vi "TCP_finding.vi"() -> ()   [LabVIEW 2018]
uses:
  <vilib>/Platform/TimedLoop/XDataNode/timing_clust.ctl
  <vilib>/Platform/TimedLoop/XDataNode/nitl_modes.ctl
  <vilib>/Platform/TimedLoop/XDataNode/wakeup.ctl
  <vilib>/Analysis/_algsub.llb/Real PseudoInverse Matrix.vi
  <vilib>/Analysis/baseanly.llb/A x Vector.vi
  <vilib>/Analysis/Matrix/Numeric/Subtract/Subtract - RM,RM.vi
  <vilib>/Platform/TimedLoop/XDataNode/XDataNode.xnode
  <vilib>/Platform/TimedLoop/XDataNode/XDNodeRunTimeDep.lvlib
  <vilib>/Analysis/Matrix/NI_Matrix.lvlib
  <vilib>/Analysis/NI_AALPro.lvlib
  <vilib>/Analysis/NI_AALBase.lvlib
panel:
  in  "Set":bool
  out "Finished Late_Monitor":u32
  out "Finished Late_Matrix":u32
  in  "stop":bool
  out "Pos 3":T1={"X"=196.167, "Y"=47.983, "Z"=275.578, "X_theta"=160.982, "Y_theta"=40.126, "Z_theta"=-130.827} {"Z_theta" format="%#_8f"; "Y_theta" format="%#_8f"; "X_theta" format="%#_8f"; "Z" format="%#_8f"; "Y" format="%#_8f"; "X" format="%#_8f"}
  out "Pos 4":T1={"X"=168.527, "Y"=22.423, "Z"=245.207, "X_theta"=177.832, "Y_theta"=63.314, "Z_theta"=-166.919} {"Z_theta" format="%#_8f"; "Y_theta" format="%#_8f"; "X_theta" format="%#_8f"; "Z" format="%#_8f"; "Y" format="%#_8f"; "X" format="%#_8f"}
  out "Pos 2":T1={"X"=193.917, "Y"=-20.843, "Z"=266.17, "X_theta"=-149.895, "Y_theta"=42.769, "Z_theta"=158.347} {"Z_theta" format="%#_8f"; "Y_theta" format="%#_8f"; "X_theta" format="%#_8f"; "Z" format="%#_8f"; "Y" format="%#_8f"; "X" format="%#_8f"}
  out "Pos 1":T1={"X"=173.917, "Y"=16.457, "Z"=254.971, "X_theta"=-176.204, "Y_theta"=57.893, "Z_theta"=-177.155} {"Z_theta" format="%#_8f"; "Y_theta" format="%#_8f"; "X_theta" format="%#_8f"; "Z" format="%#_8f"; "Y" format="%#_8f"; "X" format="%#_8f"}
  out "TCP":dbl[](array[numeric]) format="%#_4g"
  in  "find":bool
  in  "Save Pos 4":bool
  in  "Save Pos 3":bool
  in  "Save Pos 2":bool
  in  "Save Pos 1":bool
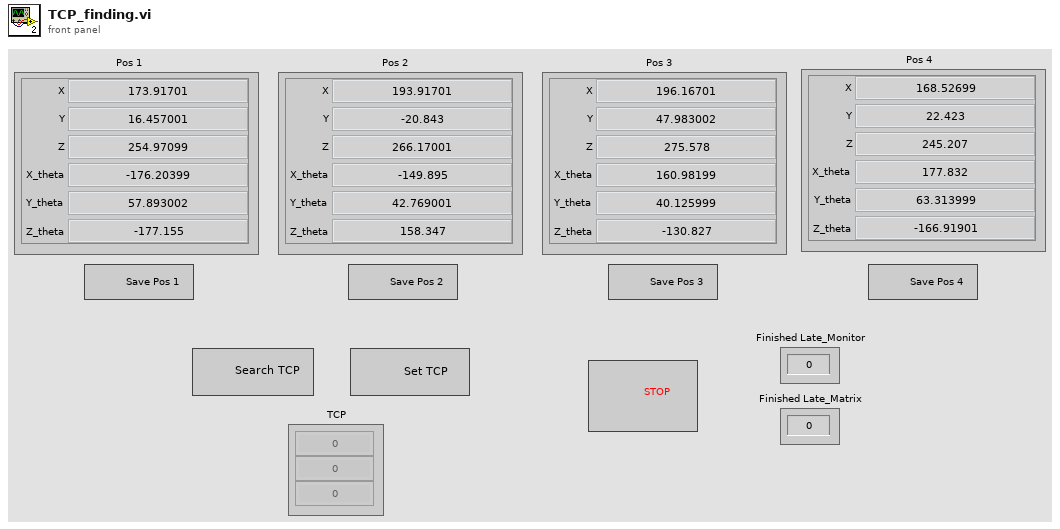
[diagram p1: front panel]
types:
  T1 = cluster{"X":sgl, "Y":sgl, "Z":sgl, "X_theta":sgl, "Y_theta":sgl, "Z_theta":sgl}
  T2 = typedef "XDNodeRunTimeDep.lvlib/timing_clust.ctl" = cluster{"Expected End [f-1]":u64, "Actual End [f-1]":u64, "Finished Late? [f-1]":bool, "Expected End [i-1]":u64, "Actual End [i-1]":u64, "Finished Late? [i-1]":bool, "Expected Start [i]":u64, "Actual Start [i]":u64, "Expected Start [f]":u64, "Actual Start [f]":u64, "Source Name":string, "Structure Name":string, "Period":i64, "Deadline":i64, "Offset":i64, "Start":i64, "Priority":i32, "Timeout":i32, "Mode":T3, "Wakeup Reason":T4, "Error":errorcluster, "Source Type":string, "Secondary Source Type":string, "Global End Time":u64, "Global Start Time":u64, "Frame Duration":u64, "Iteration Duration":u64, "Assigned CPU":i32, "I/O Scan Engine Mode":u32}
  T3 = typedef "XDNodeRunTimeDep.lvlib/nitl_modes.ctl" = enum32{"No Change", "Process missed periods, maintain original phase", "Discard missed periods, maintain original phase", "Process missed periods, ignore original phase", "Discard missed periods, ignore original phase"}
  T4 = typedef "XDNodeRunTimeDep.lvlib/wakeup.ctl" = enum32{"Normal", "Aborted", "Asynchronous wakeup", "Timing source error", "Timed loop error", "Timeout"}
  T5 = typedef "NI_Matrix.lvlib/RealMatrix.ctl" = dbl[][]
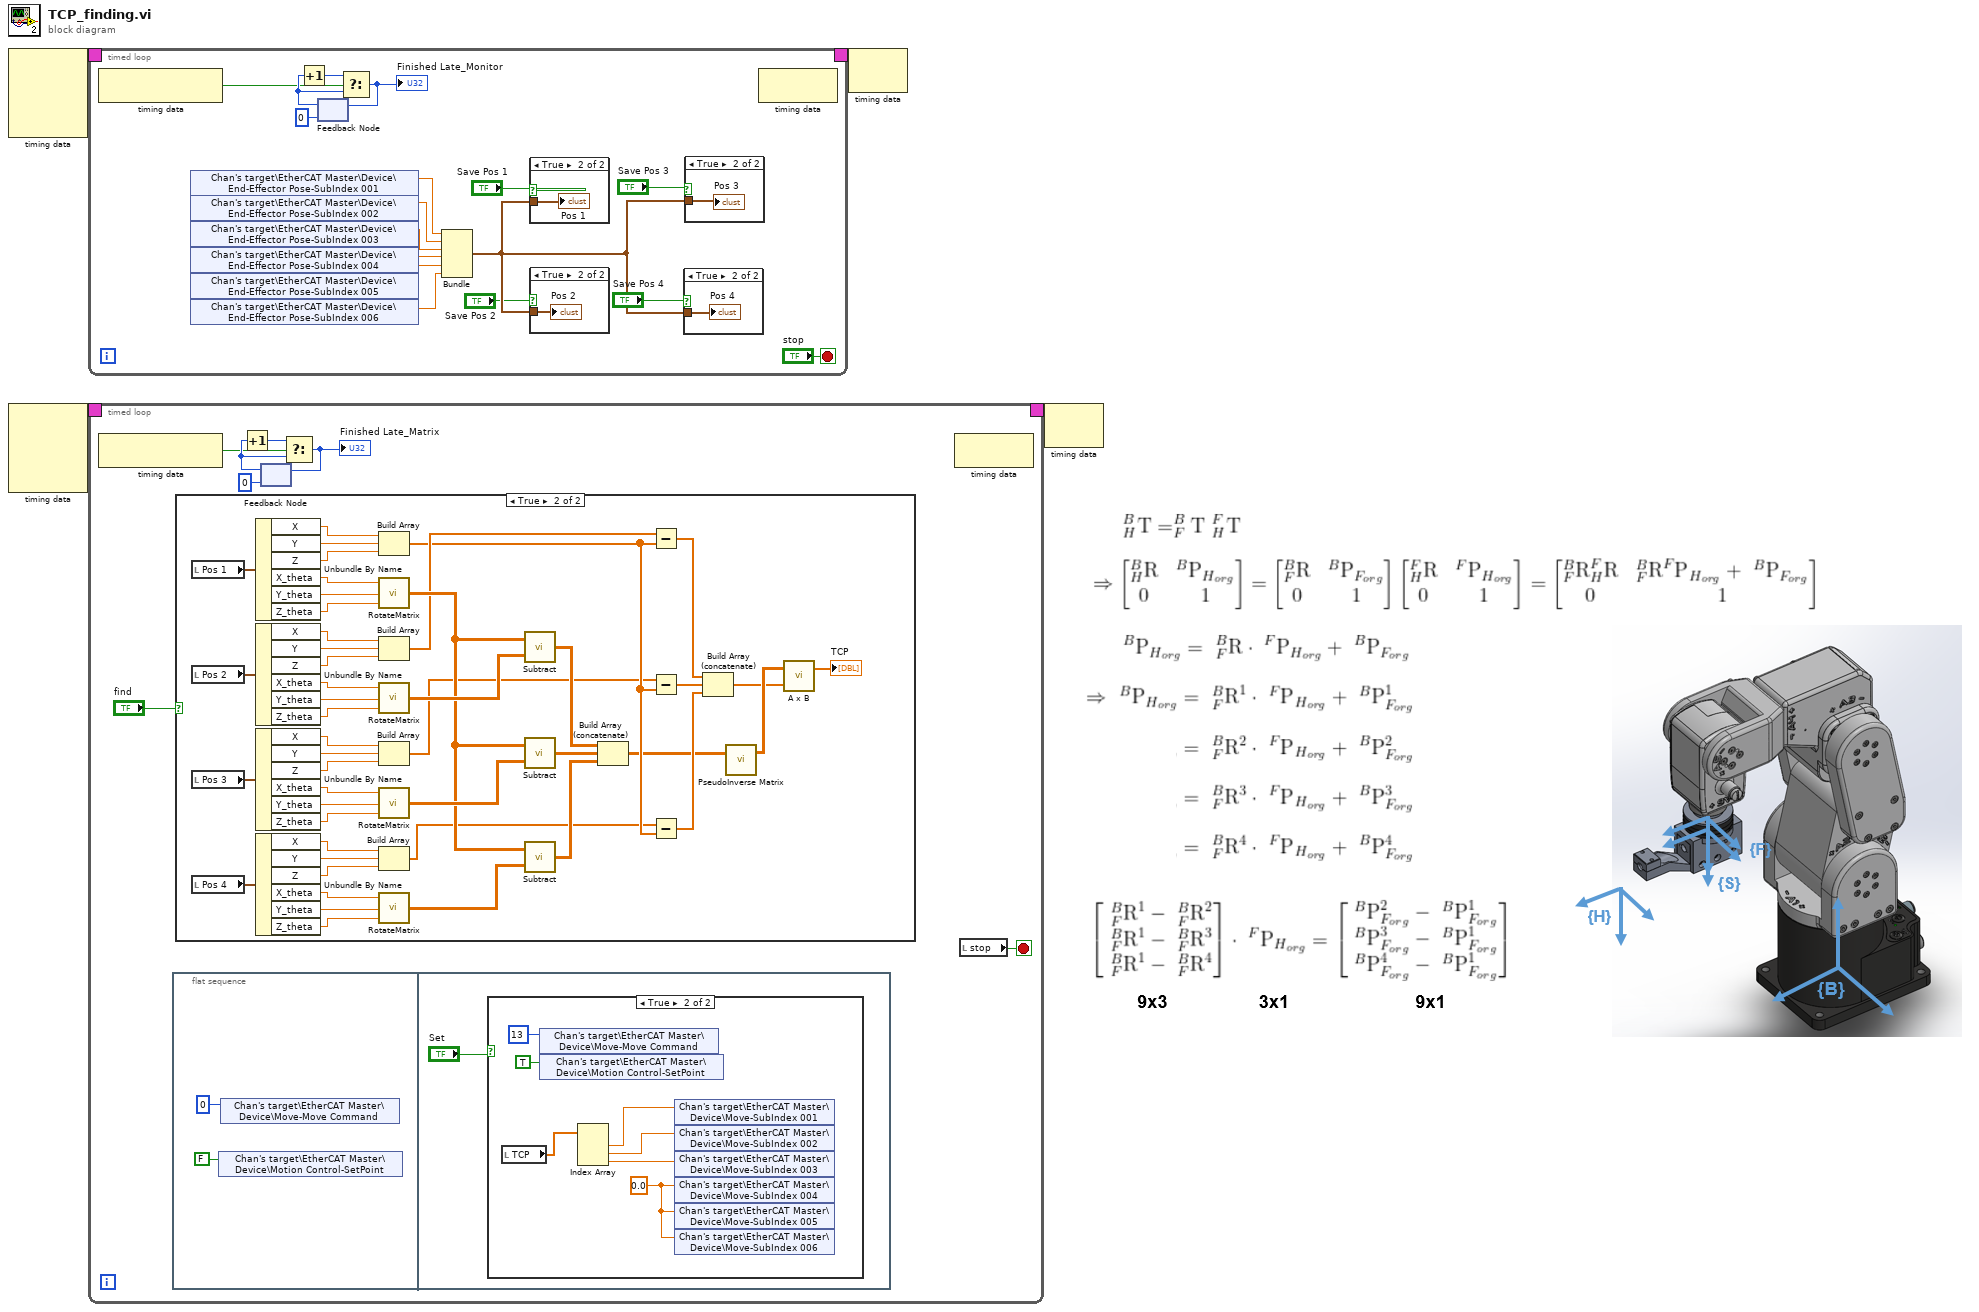
[diagram p0: block diagram]
diagram:
  n1 = node-c288() -> (w4:T2)  [unwired: 4 in]
  n2 = node-c288() -> (w2:T2)  [unwired: 4 in]
  n3 = timed-loop {
    timing: w4 -> [_]
    timing-out: [_] -> w3
    stop <- "stop" stop-if-true
    n4 = node-c288() -> (w5:bool)  [unwired: 1 in]
    n5 = shared-variable "Chan's target\\EtherCAT Master\\Device\\End-Effector Pose-SubIndex 001"() -> (w16:sgl)  [unwired: 1 in, 1 out]
    n6 = shared-variable "Chan's target\\EtherCAT Master\\Device\\End-Effector Pose-SubIndex 002"() -> (w17:sgl)  [unwired: 1 in, 1 out]
    n7 = shared-variable "Chan's target\\EtherCAT Master\\Device\\End-Effector Pose-SubIndex 003"() -> (w18:sgl)  [unwired: 1 in, 1 out]
    n8 = shared-variable "Chan's target\\EtherCAT Master\\Device\\End-Effector Pose-SubIndex 004"() -> (w19:sgl)  [unwired: 1 in, 1 out]
    n9 = shared-variable "Chan's target\\EtherCAT Master\\Device\\End-Effector Pose-SubIndex 005"() -> (w20:sgl)  [unwired: 1 in, 1 out]
    n10 = shared-variable "Chan's target\\EtherCAT Master\\Device\\End-Effector Pose-SubIndex 006"() -> (w21:sgl)  [unwired: 1 in, 1 out]
    n11 = feedback #1(u32 0) -> (w7:u32)
    n12 = Increment(x=w7) -> (x+1=w8:u32)
    n13 = Select(t=w8, s=w5, f=w7) -> (s? t:f=w9:u32)
    "Finished Late_Monitor" <- w9
    n14 = feedback-in #1(w9) -> ()
    n15 = Bundle(w16, w17, w18, w19, w20, w21) -> (w14:cluster{sgl, sgl, sgl, sgl, sgl, sgl})  [unwired: 1 in]
    n16 = case shown="True" "Save Pos 1" {
      tunnel: w14 -> [_ w25]
      frame False {
      }
      frame True {
        "Pos 1" <- w25
      }
    }
    n17 = case shown="True" "Save Pos 2" {
      tunnel: w14 -> [_ w24]
      frame False {
      }
      frame True {
        "Pos 2" <- w24
      }
    }
    n18 = case shown="True" "Save Pos 4" {
      tunnel: w14 -> [_ w23]
      frame False {
      }
      frame True {
        "Pos 4" <- w23
      }
    }
    n19 = case shown="True" "Save Pos 3" {
      tunnel: w14 -> [_ w22]
      frame False {
      }
      frame True {
        "Pos 3" <- w22
      }
    }
    n20 = node-c288() -> ()  [unwired: 1 in, 1 out]
  }
  n21 = timed-loop {
    timing: w2 -> [_]
    timing-out: [_] -> w1
    stop <- w34 stop-if-true
    n22 = node-c288() -> (w29:bool)  [unwired: 1 in]
    n23 = flat-sequence {
      frame #0 {
        n24 = shared-variable "Chan's target\\EtherCAT Master\\Device\\Motion Control-SetPoint"(FALSE ("Motion Control-SetPoint")) -> ()  [unwired: 1 in, 1 out]
        n25 = shared-variable "Chan's target\\EtherCAT Master\\Device\\Move-Move Command"(u32 0 ("Move-Move Command")) -> ()  [unwired: 1 in, 1 out]
      }
      frame #1 {
        n26 = case shown="True" "Set" {
          frame False {
          }
          frame True {
            w39 = sgl 0.0 ("Move-SubIndex 004")
            n27 = local read "TCP"() -> (w43:dbl[])
            n28 = shared-variable "Chan's target\\EtherCAT Master\\Device\\Move-Move Command"(u32 13 ("Move-Move Command")) -> ()  [unwired: 1 in, 1 out]
            n29 = shared-variable "Chan's target\\EtherCAT Master\\Device\\Motion Control-SetPoint"(TRUE ("Motion Control-SetPoint")) -> ()  [unwired: 1 in, 1 out]
            n30 = Index Array(array=w43) -> (element #1=w42:dbl, element #2=w41:dbl, element #3=w40:dbl)  [unwired: 3 in]
            n31 = shared-variable "Chan's target\\EtherCAT Master\\Device\\Move-SubIndex 001"(w42) -> ()  [unwired: 1 in, 1 out]
            n32 = shared-variable "Chan's target\\EtherCAT Master\\Device\\Move-SubIndex 002"(w41) -> ()  [unwired: 1 in, 1 out]
            n33 = shared-variable "Chan's target\\EtherCAT Master\\Device\\Move-SubIndex 003"(w40) -> ()  [unwired: 1 in, 1 out]
            n34 = shared-variable "Chan's target\\EtherCAT Master\\Device\\Move-SubIndex 004"(w39) -> ()  [unwired: 1 in, 1 out]
            n35 = shared-variable "Chan's target\\EtherCAT Master\\Device\\Move-SubIndex 005"(w39) -> ()  [unwired: 1 in, 1 out]
            n36 = shared-variable "Chan's target\\EtherCAT Master\\Device\\Move-SubIndex 006"(w39) -> ()  [unwired: 1 in, 1 out]
          }
        }
      }
    }
    n37 = case shown="True" "find" {
      frame False {
      }
      frame True {
        n38 = local read "Pos 1"() -> (w91:T1)
        n39 = local read "Pos 2"() -> (w78:T1)
        n40 = local read "Pos 3"() -> (w65:T1)
        n41 = local read "Pos 4"() -> (w64:T1)
        n42 = Unbundle By Name(w91) -> ("X"=w90:sgl, "Y"=w89:sgl, "Z"=w88:sgl, "X_theta"=w87:sgl, "Y_theta"=w86:sgl, "Z_theta"=w85:sgl)
        n43 = Unbundle By Name(w78) -> ("X"=w84:sgl, "Y"=w83:sgl, "Z"=w82:sgl, "X_theta"=w81:sgl, "Y_theta"=w80:sgl, "Z_theta"=w79:sgl)
        n44 = Unbundle By Name(w65) -> ("X"=w77:sgl, "Y"=w76:sgl, "Z"=w75:sgl, "X_theta"=w74:sgl, "Y_theta"=w73:sgl, "Z_theta"=w72:sgl)
        n45 = Unbundle By Name(w64) -> ("X"=w71:sgl, "Y"=w70:sgl, "Z"=w69:sgl, "X_theta"=w68:sgl, "Y_theta"=w67:sgl, "Z_theta"=w66:sgl)
        n46 = Build Array(w90, w89, w88) -> (w55:sgl[])
        n47 = call "RotateMatrix.vi"("gamma"=w85, "beta"=w86, "alpha"=w87) -> ("Rotate Matrix"=w61:T5)
        n48 = Build Array(w84, w83, w82) -> (w56:sgl[])
        n49 = call "RotateMatrix.vi"("gamma"=w79, "beta"=w80, "alpha"=w81) -> ("Rotate Matrix"=w63:T5)
        n50 = Build Array(w77, w76, w75) -> (w53:sgl[])
        n51 = call "RotateMatrix.vi"("gamma"=w72, "beta"=w73, "alpha"=w74) -> ("Rotate Matrix"=w62:T5)
        n52 = Build Array(w71, w70, w69) -> (w54:sgl[])
        n53 = call "RotateMatrix.vi"("gamma"=w66, "beta"=w67, "alpha"=w68) -> ("Rotate Matrix"=w60:T5)
        n54 = call-poly <vilib>:"Subtract.vi"("Real Matrix B"=w63, "Real Matrix A"=w61) -> ("A - B"=w59:T5)
        n55 = call-poly <vilib>:"Subtract.vi"("Real Matrix B"=w62, "Real Matrix A"=w61) -> ("A - B"=w58:T5)
        n56 = call-poly <vilib>:"Subtract.vi"("Real Matrix B"=w60, "Real Matrix A"=w61) -> ("A - B"=w57:T5)
        n57 = Build Array (concatenate)(w59, w58, w57) -> (w49:T5)
        n58 = Subtract ("Subtract.vi")(x=w56, y=w55) -> (x-y=w52:sgl[])
        n59 = Subtract ("Subtract.vi")(x=w53, y=w55) -> (x-y=w51:sgl[])
        n60 = Subtract ("Subtract.vi")(x=w54, y=w55) -> (x-y=w50:sgl[])
        n61 = Build Array (concatenate)(w52, w51, w50) -> (w47:sgl[])
        n62 = call-poly <vilib>:"PseudoInverse Matrix.vi"("Input Matrix"=w49) -> ("PseudoInverse Matrix"=w48:T5)  [unwired: 1 in, 1 out]
        n63 = call-poly <vilib>:"A x B.vi"("Vector"=w47, "A"=w48) -> ("A x Vector"=→"TCP":dbl[])  [unwired: 1 out]
      }
    }
    n64 = feedback #2(u32 0) -> (w31:u32)
    n65 = Increment(x=w31) -> (x+1=w32:u32)
    n66 = Select(t=w32, s=w29, f=w31) -> (s? t:f=w33:u32)
    "Finished Late_Matrix" <- w33
    n67 = feedback-in #2(w33) -> ()
    n68 = node-c288() -> ()  [unwired: 1 in, 1 out]
    n69 = local read "stop"() -> (w34:bool)
  }
  n70 = node-c288(w3) -> ()  [unwired: 1 out]
  n71 = node-c288(w1) -> ()  [unwired: 1 out]
